vi "basic com port send response test.vi"(0 "VISA Send port":refnum<visa-resource-name>, 1 "Expected response":string, 2 "VISA Response Port":refnum<visa-resource-name>, 5 "Baud":dbl=115200.0, 7 "Open serial comm port (F)?":bool, 9 "Send text":string, 11 "error in (no error)":errorcluster, 12 "Wait for response msecs":dbl=750.0, 13 "Comparison type":T1=enum."String in response somewhere") -> (4 "Response valid?":bool, 6 "Response":string, 8 "VISA Send port out":refnum<visa-resource-name>, 10 "VISA Response Port out":refnum<visa-resource-name>, 15 "error out":errorcluster)   [LabVIEW 2013]
uses:
  Test Support VI/String compare type.ctl
panel:
  out "Bytes at port":u32
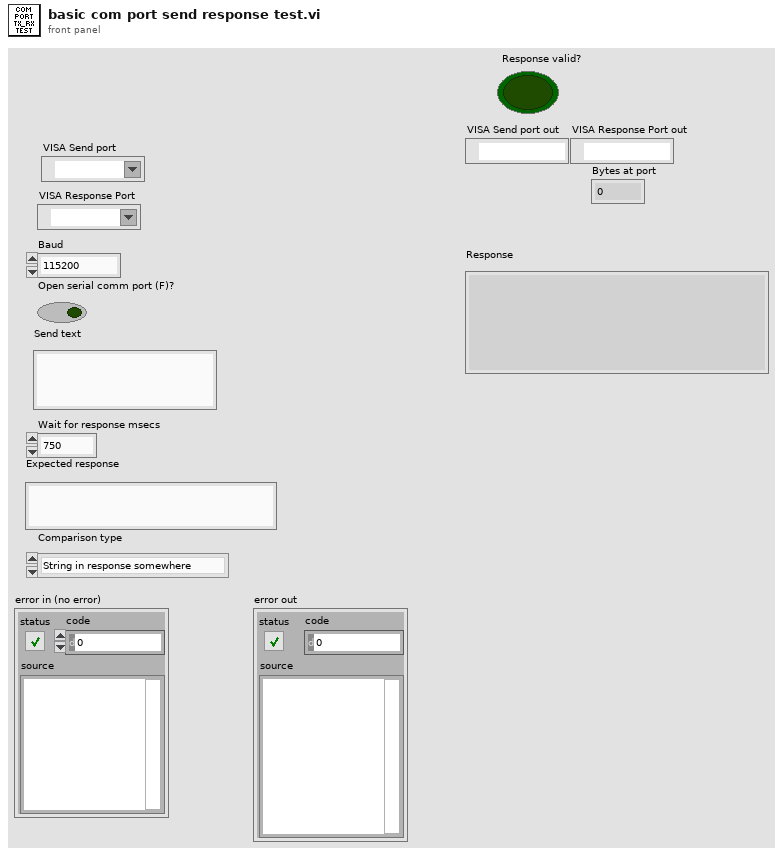
[diagram p1: front panel]
types:
  T1 = typedef "String compare type.ctl" = enum16{"String is exactly response", "String in response somewhere", "String not in response"}
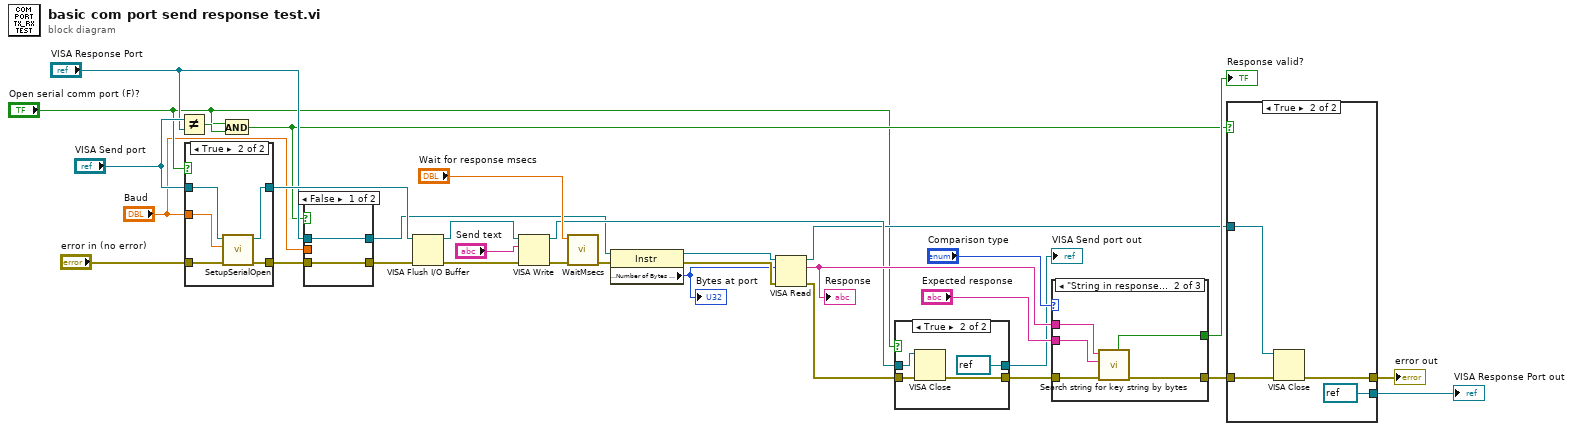
[diagram p0: block diagram]
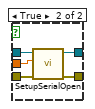
[diagram p3: hidden frame]
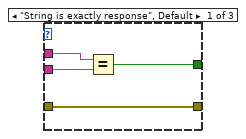
[diagram p5: hidden frame]
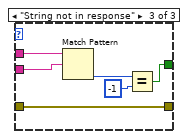
[diagram p6: hidden frame]
diagram:
  n1 = Not Equal?(x="VISA Send port", y="VISA Response Port") -> (x != y?=w10:bool)
  n2 = case shown="True" "Open serial comm port (F)?" {
    tunnel: "error in (no error)" -> [w33 w39]
    tunnel: "VISA Send port" -> [w34 w38]
    tunnel: "Baud" -> [_ w37]
    tunnel: [w33 w36] -> w15
    tunnel: [w34 w35] -> w32
    frame False {
    }
    frame True {
      n3 = call "SetupSerialOpen.vi"("error in (no error)"=w39, "Baud"=w37, "VISA Refnum in"=w38) -> ("error out"=w36:errorcluster, "VISA session"=w35:refnum<visa-resource-name>)  [unwired: 7 in]
    }
  }
  n4 = And(x="Open serial comm port (F)?", y=w10) -> (x .and. y?=w6:bool)
  n5 = case shown="False" w6 {
    tunnel: w15 -> [w40 w46]
    tunnel: "VISA Response Port" -> [w41 w45]
    tunnel: "Baud" -> [_ w44]
    tunnel: [w40 w43] -> w14
    tunnel: [w41 w42] -> w13
    frame False {
    }
    frame True {
      n6 = call "SetupSerialOpen.vi"("error in (no error)"=w46, "Baud"=w44, "VISA Refnum in"=w45) -> ("error out"=w43:errorcluster, "VISA session"=w42:refnum<visa-resource-name>)  [unwired: 7 in]
    }
  }
  n7 = VISA Flush I/O Buffer(VISA resource name=w32, error in (no error)=w14) -> (VISA resource name out=w30:refnum<visa-resource-name>, error out=w31:errorcluster)  [unwired: 1 in]
  n8 = VISA Write(VISA resource name=w30, write buffer="Send text", error in (no error)=w31) -> (VISA resource name out=w16:refnum<visa-resource-name>, error out=w28:errorcluster)  [unwired: 1 out]
  n9 = call "WaitMsecs.vi"("error in (no error)"=w28, "Wait Msecs"="Wait for response msecs") -> ("error out"=w26:errorcluster)  [unwired: 9 in]
  n10 = property class="Instr"(reference=w13, error in=w26) -> (reference out=w23:refnum<visa-resource-name>, error out=w25:errorcluster, "Serial Settings:Number of Bytes at Serial Port"=w24:u32)
  "Bytes at port" <- w24
  n11 = VISA Read(VISA resource name=w23, byte count=w24, error in (no error)=w25) -> (VISA resource name out=w9:refnum<visa-resource-name>, read buffer=w21:string, error out=w20:errorcluster)  [unwired: 1 out]
  "Response" <- w21
  n12 = case shown="True" "Open serial comm port (F)?" {
    tunnel: w16 -> [w47 w52]
    tunnel: w20 -> [w48 w51]
    tunnel: [w48 w50] -> w19
    tunnel: [w47 refnum<visa-resource-name> refnum ("VISA session")] -> w2
    frame False {
    }
    frame True {
      n13 = VISA Close(VISA resource name=w52, error in (no error)=w51) -> (error out=w50:errorcluster)
    }
  }
  "VISA Send port out" <- w2
  n14 = case shown="\"String in response somewhere\"" "Comparison type" {
    tunnel: w21 -> [w56 w61 w65]
    tunnel: w19 -> [w53 w59 w62]
    tunnel: "Expected response" -> [w55 w60 w64]
    tunnel: [w54 w58 w63] -> w17
    tunnel: [w53 w57 w62] -> w7
    frame "String is exactly response", Default {
      n15 = Equal?(x=w56, y=w55) -> (x = y?=w54:bool)
    }
    frame "String in response somewhere" {
      n16 = call "Search string for key string by bytes.vi"("error in (no error)"=w59, "Search for string"=w60, "String"=w61) -> ("error out"=w57:errorcluster, "Found match?"=w58:bool)  [unwired: 4 in, 3 out]
    }
    frame "String not in response" {
      n17 = Match Pattern(string=w65, regular expression=w64) -> (offset past match=w67:i32)  [unwired: 1 in, 3 out]
      n18 = Equal?(x=w67, y=-1) -> (x = y?=w63:bool)
    }
  }
  "Response valid?" <- w17
  n19 = case shown="True" w6 {
    tunnel: w9 -> [w68 w73]
    tunnel: [w69 w72] -> w8
    tunnel: w7 -> [w69 w71]
    tunnel: [w68 refnum<visa-resource-name> refnum ("VISA session")] -> w1
    frame False {
    }
    frame True {
      n20 = VISA Close(VISA resource name=w73, error in (no error)=w71) -> (error out=w72:errorcluster)
    }
  }
  "error out" <- w8
  "VISA Response Port out" <- w1
